vi "CgHandShapes.vi"() -> ()   [LabVIEW 2009]
uses:
  <vilib>/Utility/file.llb/Write To Spreadsheet File (DBL).vi
panel:
  out "RH Degrees":dbl[](array[numeric])
  out "LH Degrees":dbl[](array[numeric])
  in  "stop":bool
  in  "Collect":bool
  out "LH Cal Warning":bool
  out "RH Cal Warning":bool
  in  "RH Calibration":string="RH_Calibration1.cal"
  in  "LH Calibration":string="LH_Calibration1.cal"
  in  "Subject Initials":string="Default"
  in  "LH COM Port":refnum<visa-resource-name>="COM1"
  in  "RH COM Port":refnum<visa-resource-name>="COM2"
  out "Sensor Names":string[](array[string])
  # "(Pg Down)"
  # "(Pg Up)"
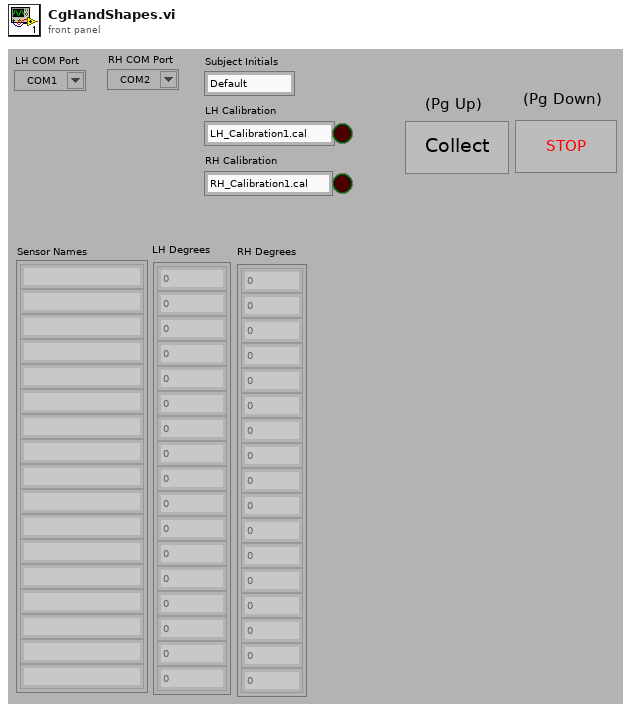
[diagram p1: front panel]
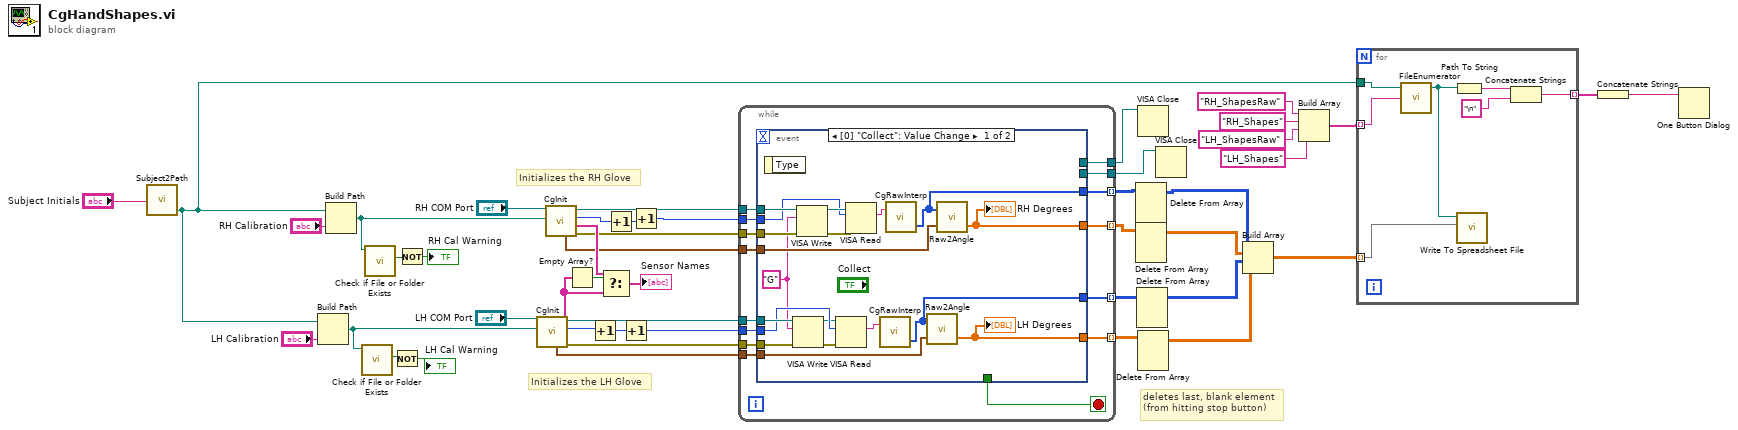
[diagram p0: block diagram]
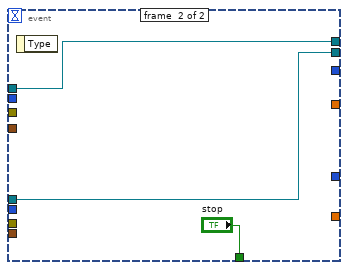
[diagram p2: hidden frame]
diagram:
  # "deletes last, blank element\n(from hitting stop button)"
  # "Initializes the LH Glove"
  # "Initializes the RH Glove"
  n1 = call "Subject2Path.vi"("Subject Initials"="Subject Initials") -> ("Calibration Path"=w3:path)  [unwired: 1 in, 2 out]
  n2 = Build Path(base path=w3, name or relative path="LH Calibration") -> (appended path=w34:path)
  n3 = Build Path(base path=w3, name or relative path="RH Calibration") -> (appended path=w38:path)
  n4 = call <vilib>:"Check if File or Folder Exists.vi"("path"=w34) -> ("file or folder exists?"=w33:bool)  [unwired: 8 in, 2 out]
  n5 = call <vilib>:"Check if File or Folder Exists.vi"("path"=w38) -> ("file or folder exists?"=w37:bool)  [unwired: 8 in, 2 out]
  n6 = Not(x=w33) -> (.not. x?=→"LH Cal Warning":bool)
  n7 = Not(x=w37) -> (.not. x?=→"RH Cal Warning":bool)
  n8 = call "CgInit.vi"("Calibration File"=w34, "VISA resource name"="LH COM Port") -> ("error out"=w26:errorcluster, "Sensor Names"=w43:string[], "#Sensors"=w21:i32, "VISA resource name out"=w27:refnum<visa-resource-name>, "Calibration Array"=w30:cluster{"Offset":dbl, "Gain":dbl}[])  [unwired: 3 in]
  n9 = call "CgInit.vi"("Calibration File"=w38, "VISA resource name"="RH COM Port") -> ("error out"=w28:errorcluster, "Sensor Names"=w46:string[], "#Sensors"=w24:i32, "VISA resource name out"=w29:refnum<visa-resource-name>, "Calibration Array"=w31:cluster{"Offset":dbl, "Gain":dbl}[])  [unwired: 3 in]
  n10 = Empty Array?(array=w43) -> (empty?=w45:bool)
  n11 = Increment(x=w21) -> (x+1=w25:i32)
  n12 = Select(t=w46, s=w45, f=w43) -> (s? t:f=→"Sensor Names":string[])
  n13 = Increment(x=w24) -> (x+1=w23:i32)
  n14 = Increment(x=w25) -> (x+1=w20:i32)
  n15 = Increment(x=w23) -> (x+1=w22:i32)
  n16 = while {
    tunnel: w31 -> [w61]
    tunnel: w30 -> [w60]
    tunnel: w29 -> [w59]
    tunnel: w28 -> [w58]
    tunnel: w27 -> [w57]
    tunnel: w26 -> [w56]
    tunnel: w22 -> [w55]
    tunnel: w20 -> [w54]
    tunnel: [w53] -> w15
    tunnel: [w52] -> w14
    tunnel: [w51] -> w17 mode=indexing
    tunnel: [w50] -> w16 mode=indexing
    tunnel: [w48] -> w19 mode=indexing
    tunnel: [w47] -> w18 mode=indexing
    stop <- w49 stop-if-true
    n17 = event shown="[0] \"Collect\": Value Change" {
      selector: _ -> [_ _]
      dyn-events: _ -> [_ _]
      timeout: _ -> [_ _]
      tunnel: w61 -> [w80 _]
      tunnel: w60 -> [w79 _]
      tunnel: w59 -> [w78 w81]
      tunnel: w58 -> [w75 _]
      tunnel: w57 -> [w74 w82]
      tunnel: w56 -> [w73 _]
      tunnel: w55 -> [w76 _]
      tunnel: w54 -> [w71 _]
      tunnel: [_ w81] -> w53
      tunnel: [_ w82] -> w52
      tunnel: [w65 _] -> w51
      tunnel: [w64 _] -> w50
      tunnel: [_ "stop"] -> w49
      tunnel: [w63 _] -> w48
      tunnel: [w62 _] -> w47
      event #0 {
        w66 = "G" ("write buffer")
        n18 = event-data() -> ()  [unwired: 1 in, 1 out]
        n19 = VISA Write(VISA resource name=w74, write buffer=w66, error in (no error)=w73) -> (VISA resource name out=w70:refnum<visa-resource-name>, error out=w72:errorcluster)  [unwired: 1 out]
        n20 = VISA Write(VISA resource name=w78, write buffer=w66, error in (no error)=w75) -> (VISA resource name out=w77:refnum<visa-resource-name>, error out=w69:errorcluster)  [unwired: 1 out]
        n21 = VISA Read(VISA resource name=w70, byte count=w71, error in (no error)=w72) -> (read buffer=w68:string)  [unwired: 3 out]
        n22 = VISA Read(VISA resource name=w77, byte count=w76, error in (no error)=w69) -> (read buffer=w67:string)  [unwired: 3 out]
        n23 = call "CgRawInterp.vi"("Cyberglove Out"=w68) -> ("Raw Data"=w65:u8[])  [unwired: 1 in, 1 out]
        n24 = call "CgRawInterp.vi"("Cyberglove Out"=w67) -> ("Raw Data"=w63:u8[])  [unwired: 1 in, 1 out]
        n25 = call "Raw2Angle.vi"("Calibration"=w79, "Raw Data"=w65) -> ("Degrees"=w64:dbl[])  [unwired: 1 out]
        "LH Degrees" <- w64
        n26 = call "Raw2Angle.vi"("Calibration"=w80, "Raw Data"=w63) -> ("Degrees"=w62:dbl[])  [unwired: 1 out]
        "RH Degrees" <- w62
      }
      event #1 {
        n27 = event-data() -> ()  [unwired: 1 in, 1 out]
      }
    }
  }
  n28 = Delete From Array(array=w19) -> (array with subset deleted=w13:u8[][])  [unwired: 3 in, 1 out]
  n29 = Delete From Array(array=w18) -> (array with subset deleted=w12:dbl[][])  [unwired: 3 in, 1 out]
  n30 = Delete From Array(array=w17) -> (array with subset deleted=w11:u8[][])  [unwired: 3 in, 1 out]
  n31 = VISA Close(VISA resource name=w15) -> ()  [unwired: 1 in, 1 out]
  n32 = Delete From Array(array=w16) -> (array with subset deleted=w10:dbl[][])  [unwired: 3 in, 1 out]
  n33 = VISA Close(VISA resource name=w14) -> ()  [unwired: 1 in, 1 out]
  n34 = Build Array(w13, w12, w11, w10) -> (w4:dbl[][][])
  n35 = Build Array("RH_ShapesRaw" ("write buffer"), "RH_Shapes" ("write buffer"), "LH_ShapesRaw" ("write buffer"), "LH_Shapes" ("write buffer")) -> (w5:string[])
  n36 = for {
    tunnel: w5 -> [w89] mode=indexing
    tunnel: w4 -> [w88] mode=indexing
    tunnel: w3 -> [w90]
    tunnel: [w84] -> w2 mode=indexing
    n37 = call "FileEnumerator.vi"("Filename"=w89, "Path"=w90) -> ("appended path"=w87:path)  [unwired: 1 in, 2 out]
    n38 = Path To String(path=w87) -> (string=w86:string)
    n39 = call-poly <vilib>:"Write To Spreadsheet File.vi"("2D data"=w88, "file path (dialog if empty)"=w87) -> ()  [unwired: 6 in, 1 out]
    n40 = Concatenate Strings(w86, "\n" ("write buffer")) -> (w84:string)
  }
  n41 = Concatenate Strings(w2) -> (w1:string)
  n42 = One Button Dialog(message=w1) -> ()  [unwired: 1 in, 1 out]
